vi "Send Local message.vi"(6 "ok message":string, 7 "object":string="AZ1", 8 "error in (no error)":errorcluster, 9 "message header":string, 10 "header":string, 11 "messages":refnum<queue>) -> (0 "error out":errorcluster)   [LabVIEW 2019]
uses:
  Messages/ctl/LocalMsg.ctl
  table name.vi
  compress_messages.vi
  Timer Delay/format datetime 100ms.vi
  Messages/Messages.lvlib
  Alarms/Alarms.lvlib
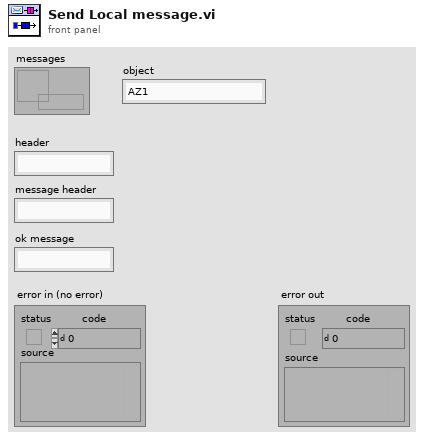
[diagram p1: front panel]
types:
  T1 = typedef "Messages.lvlib/LocalMsg.ctl" = cluster{"time stamp":timestamp, "object":string, "header":string, "message":string}
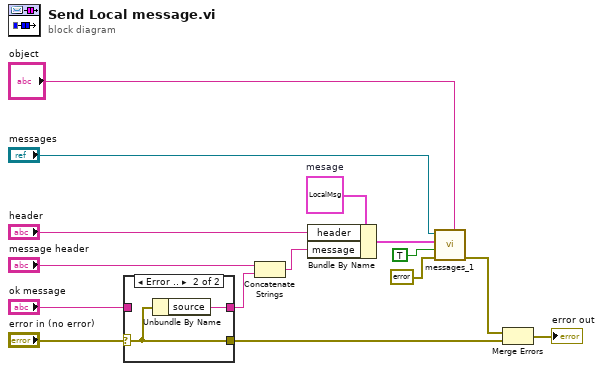
[diagram p0: block diagram]
diagram:
  w10 = T1 {"time stamp"=timestamp(0 s since 1904-01-01), "object"="", "header"="", "message"=""}  # mesage
  n1 = case shown="Error .." "error in (no error)" {
    selector: "error in (no error)" -> [w16 w18]
    tunnel: [w17 w19] -> w13
    tunnel: "ok message" -> [w17 _]
    tunnel: [w16 w18] -> w7
    frame No Error {
    }
    frame Error {
      n2 = Unbundle By Name(w18) -> ("source"=w19:string)
    }
  }
  n3 = Concatenate Strings("message header", w13) -> (w14:string)
  n4 = Bundle By Name(cluster=w10, "header"="header", "message"=w14) -> (w6:T1)
  n5 = call "messages_1.vi"("object"="object", "error in (no error)"=errorcluster {"status"=FALSE, "code"=0, "source"=""}, "Data to write (no data)"=TRUE, "mesage"=w6, "messages"="messages") -> ("error out"=w4:errorcluster)  [unwired: 5 in, 1 out]
  n6 = Merge Errors(w4, w7) -> (→"error out":errorcluster)
